vi "Initialize.vi"(5 "components directory (default)":path, 7 "framework options":T1, 8 "error in (no error)":errorcluster, 10 "framework configuration":T6, 11 "Framework in":refnum<class "Framework.lvclass">) -> (0 "error out":errorcluster, 3 "Framework out":refnum<class "Framework.lvclass">)   [LabVIEW 2017, in "DSF Core.lvlib" / "Framework.lvclass"]
uses:
  Framework.lvclass
  Thread/Plugin/Plugin Thread.lvclass
  C:/Git/DSF/Data Sharing Framework/Source/Core/Classes/Thread/Thread.lvclass
  Dispatcher/Dispatcher Thread.lvclass
  Typedefs/DSF Timing Info.ctl
  DSF Core.lvlib
  Typedefs/DSF Direction.ctl
  Typedefs/DSF Byte Order.ctl
  Typedefs/DSF Data Type.ctl
  Typedefs/DSF Settings Info.ctl
  Typedefs/DSF Engine Channel Configuration.ctl
  Typedefs/DSF Engine Transfer Configuration.ctl
  Typedefs/DSF Engine Transfer Group Configuration.ctl
  Typedefs/DSF Engine Plugin Configuration.ctl
  Typedefs/DSF Engine Framework Configuration.ctl
  Typedefs/DSF FIFO Options.ctl
  Thread/DSF Thread Options.ctl
  Framework Options.ctl
  Typedefs/DSF Plugin Options.ctl
  Typedefs/DSF Engine Plugin Thread Configuration.ctl
  Typedefs/DSF Timeout Behavior.ctl
  Typedefs/DSF Performance Options.ctl
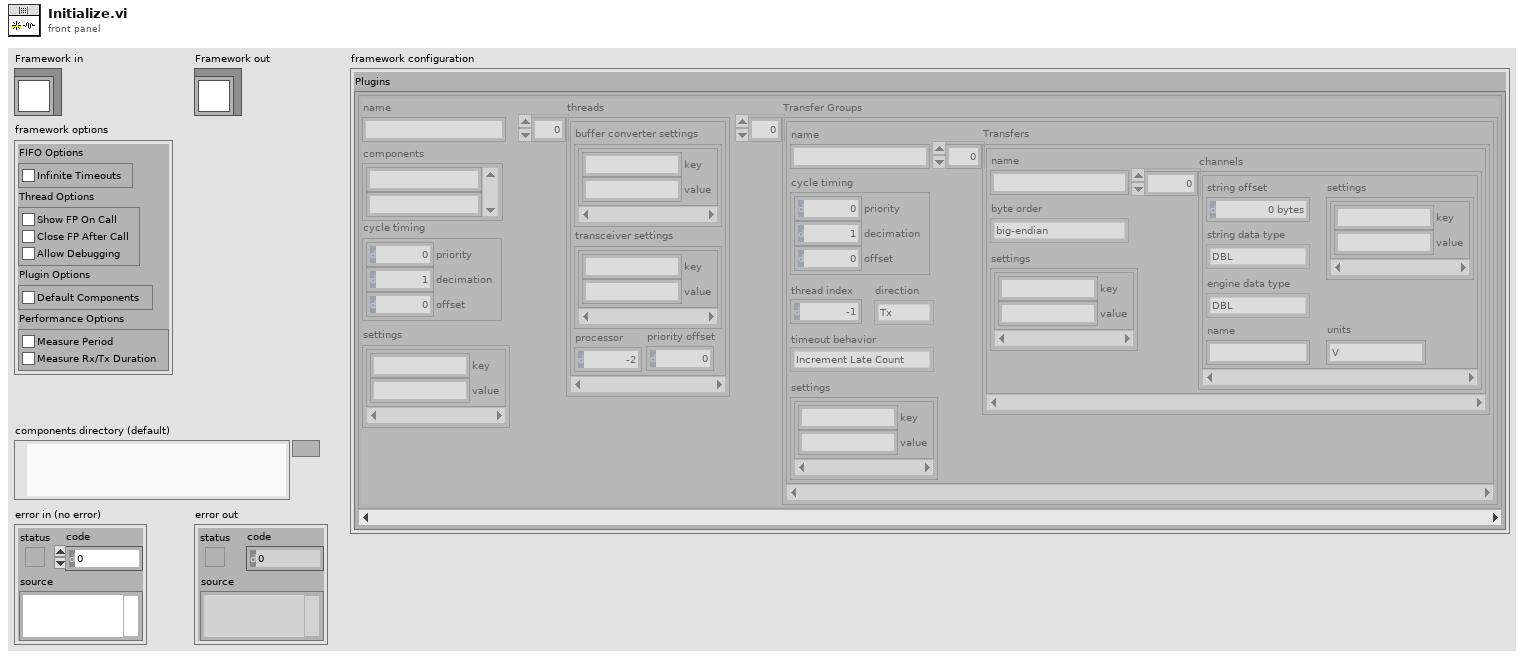
[diagram p1: front panel]
types:
  T1 = typedef "DSF Core.lvlib/Framework.lvclass/Framework Options.ctl" = cluster{"FIFO Options":T2, "Thread Options":T3, "Plugin Options":T4, "Performance Options":T5}
  T2 = typedef "DSF Core.lvlib/DSF FIFO Options.ctl" = cluster{"Infinite Timeouts":bool}
  T3 = typedef "DSF Core.lvlib/DSF Thread Options.ctl" = cluster{"Show FP On Call":bool, "Close FP After Call":bool, "Allow Debugging":bool}
  T4 = typedef "DSF Core.lvlib/DSF Plugin Options.ctl" = cluster{"Default Components":bool}
  T5 = typedef "DSF Core.lvlib/DSF Performance Options.ctl" = cluster{"Measure Period":bool, "Measure Rx/Tx Duration":bool}
  T6 = typedef "DSF Core.lvlib/DSF Engine Framework Configuration.ctl" = cluster{"Plugins":T7[]}
  T7 = typedef "DSF Core.lvlib/DSF Engine Plugin Configuration.ctl" = cluster{"name":string, "components":string[], "cycle timing":T8, "threads":T9[], "Transfer Groups":T11[], "settings":T10}
  T8 = typedef "DSF Core.lvlib/DSF Timing Info.ctl" = cluster{"priority":u64, "decimation":u64, "offset":u64}
  T9 = typedef "DSF Core.lvlib/DSF Engine Plugin Thread Configuration.ctl" = cluster{"buffer converter settings":T10, "transceiver settings":T10, "processor":i32, "priority offset":i16}
  T10 = typedef "DSF Core.lvlib/DSF Settings Info.ctl" = cluster{"key":string, "value":string}[]
  T11 = typedef "DSF Core.lvlib/DSF Engine Transfer Group Configuration.ctl" = cluster{"name":string, "direction":T12, "cycle timing":T8, "thread index":i32, "settings":T10, "Transfers":T13[], "timeout behavior":T17}
  T12 = typedef "DSF Core.lvlib/DSF Direction.ctl" = enum8{"Tx", "Rx"}
  T13 = typedef "DSF Core.lvlib/DSF Engine Transfer Configuration.ctl" = cluster{"name":string, "byte order":T14, "settings":T10, "channels":T15[]}
  T14 = typedef "DSF Core.lvlib/DSF Byte Order.ctl" = enum8{"big-endian", "little-endian"}
  T15 = typedef "DSF Core.lvlib/DSF Engine Channel Configuration.ctl" = cluster{"string offset":u64, "string data type":T16, "engine data type":T16, "name":string, "settings":T10, "units":string}
  T16 = typedef "DSF Core.lvlib/DSF Data Type.ctl" = enum8{"Bool", "SGL", "DBL", "I8", "I16", "I32", "I64", "U8", "U16", "U32", "U64"}
  T17 = typedef "DSF Core.lvlib/DSF Timeout Behavior.ctl" = enum8{"Increment Late Count", "Throw Error"}
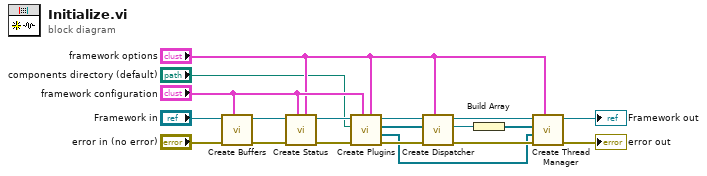
[diagram p0: block diagram]
diagram:
  n1 = call "Create Buffers.vi"("framework configuration"="framework configuration", "error in (no error)"="error in (no error)", "Framework in"="Framework in") -> ("error out"=w11:errorcluster, "Framework out"=w12:refnum<class "Framework.lvclass">)  [unwired: 7 in]
  n2 = call "Create Status.vi"("framework options"="framework options", "Framework Configuration"="framework configuration", "error in (no error)"=w11, "Framework in"=w12) -> ("error out"=w10:errorcluster, "Framework out"=w9:refnum<class "Framework.lvclass">)  [unwired: 6 in]
  n3 = call "Create Plugins.vi"("framework options"="framework options", "framework configuration"="framework configuration", "error in (no error)"=w10, "components directory"="components directory (default)", "Framework in"=w9) -> ("error out"=w18:errorcluster, "Plugin Threads"=w3:refnum<class "Plugin Thread.lvclass">[], "Plugins"=w15:refnum<class "Plugin.lvclass">[], "Framework out"=w19:refnum<class "Framework.lvclass">)  [unwired: 3 in]
  n4 = call "Create Dispatcher.vi"("framework options"="framework options", "error in (no error)"=w18, "Plugins"=w15, "Framework in"=w19) -> ("error out"=w5:errorcluster, "Dispatcher Thread"=w13:refnum<class "Dispatcher Thread.lvclass">, "Framework out"=w8:refnum<class "Framework.lvclass">)  [unwired: 5 in]
  n5 = Build Array(w13) -> (w6:refnum<class "Dispatcher Thread.lvclass">[])
  n6 = call "Create Thread Manager.vi"("framework options"="framework options", "error in (no error)"=w5, "Plugin Threads"=w3, "Framework Threads"=w6, "Framework in"=w8) -> ("error out"=→"error out":errorcluster, "Framework out"=→"Framework out":refnum<class "Framework.lvclass">)  [unwired: 5 in]
